vi "_Clear Network 56 Error.vi"(4 "error in (no error)":errorcluster) -> (1 "error out":errorcluster)   [LabVIEW 2017, in "Multi-Loop Module Example.lvlib"]
uses:
  Multi-Loop Module Example.lvlib
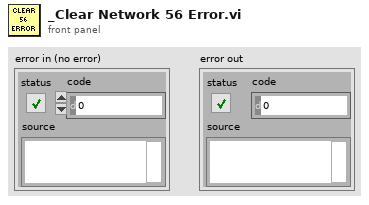
[diagram p1: front panel]
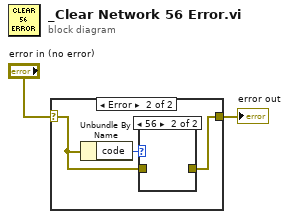
[diagram p0: block diagram]
diagram:
  n1 = case shown="Error" "error in (no error)" {
    selector: "error in (no error)" -> [w3 w5]
    tunnel: [w3 w4] -> w1
    frame No Error {
    }
    frame Error {
      n2 = Unbundle By Name(w5) -> ("code"=w6:i32)
      n3 = case shown="56" w6 {
        tunnel: w5 -> [w7 _]
        tunnel: [w7 _] -> w4
        frame Default {
        }
        frame 56 {
        }
      }
    }
  }
  "error out" <- w1
